vi "FillLocalArray.vi"(4 "Sequence Context":T1) -> (0 "error out":errorcluster, 1 "Test Data":T2 {"Numeric Measurement" format="%.2f"})   [LabVIEW 2010]
doc: "This example demonstrates how to use ActiveX to access arrays of data in TestStand from LabVIEW code modules."
uses:
  <vilib>/addons/TestStand/_TSLegacy.llb/LabVIEW Test - Test Data.ctl
  <vilib>/addons/TestStand/_TSLegacy.llb/LabVIEW Test - Sequence Context.ctl
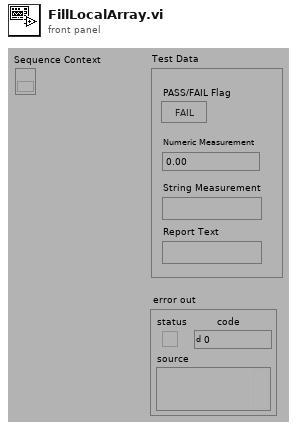
[diagram p1: front panel]
types:
  T1 = typedef "LabVIEW Test - Sequence Context.ctl" = refnum<k7>
  T2 = typedef "LabVIEW Test - Test Data.ctl" = cluster{"PASS/FAIL Flag":bool, "Numeric Measurement":dbl, "String Measurement":string, "Report Text":string}
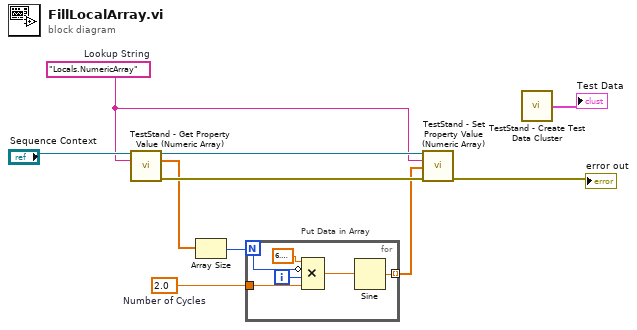
[diagram p0: block diagram]
diagram:
  w2 = 2.0  # Number of Cycles
  w4 = "Locals.NumericArray"  # Lookup String
  # "Put Data in Array"
  n1 = call <vilib>:"TestStand - Get Property Value (Numeric Array).vi"("Sequence Context In"="Sequence Context", "Lookup String"=w4) -> ("Sequence Context Out"=w6:refnum<k7>, "Value"=w5:dbl[], "error out"=w7:errorcluster)  [unwired: 1 in, 10 out]
  n2 = Array Size(array=w5) -> (size(s)=w3:i32)
  n3 = for {
    N: w3 -> [w14]
    tunnel: [w16] -> w1 mode=indexing
    tunnel: w2 -> [w12]
    i -> [w13]
    n4 = Compound Arithmetic op=MULTIPLY(6.283185307179586, invert w14, w13, w12) -> (w11:dbl)
    n5 = Sine(x=w11) -> (sin(x)=w16:dbl)
  }
  n6 = call <vilib>:"TestStand - Set Property Value (Numeric Array).vi"("Sequence Context In"=w6, "Lookup String"=w4, "New Value"=w1, "error in (no error)"=w7) -> ("error out"=→"error out":errorcluster)  [unwired: 1 in, 10 out]
  n7 = call <vilib>:"TestStand - Create Test Data Cluster.vi"() -> ("Test Data"=→"Test Data":T2)  [unwired: 4 in]
